vi "DAQ.Create DAQmx Asynch Read.vi"(8 "error in (no error)":errorcluster, 11 "Array":refnum<k21>[](array[refnum])) -> (0 "error out":errorcluster, 3 "VI out":refnum<vi>)   [LabVIEW 2019, in "Instrument.Lockin.lvlib" / "Instrument.DAQ.lvclass"]
uses:
  Instrument.DAQ.lvclass
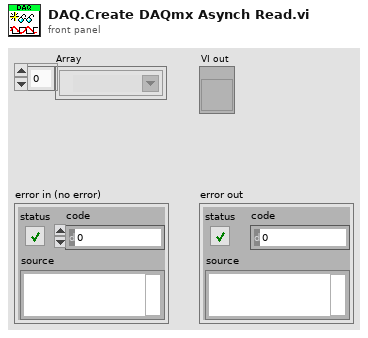
[diagram p1: front panel]
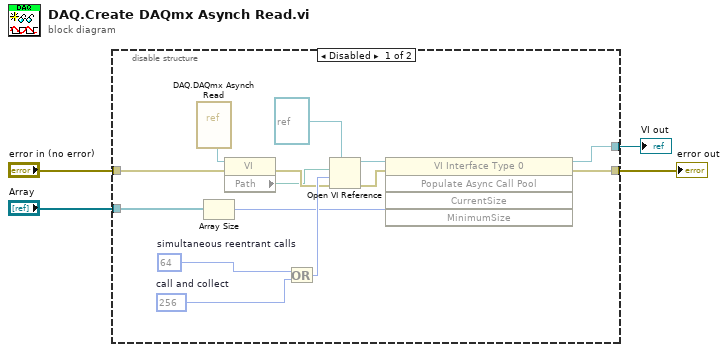
[diagram p0: block diagram]
diagram:
  n1 = disable-structure shown="Disabled" {
    disable-tunnel: "Array" -> [w8 _]
    disable-tunnel: [w7 _] -> w3
    disable-tunnel: [w6 w19] -> w2
    disable-tunnel: "error in (no error)" -> [w5 w19]
    frame Disabled {
      w16 = 64  # simultaneous reentrant calls
      w18 = 256  # call and collect
      n2 = vi-ref "DAQ.DAQmx Asynch Read.vi"() -> (w14:refnum<vi>)
      n3 = Array Size(array=w8) -> (size(s)=w15:i32)
      n4 = property class="VI"(reference=w14, error in=w5) -> (error out=w10:errorcluster, "Path"=w9:path)  [unwired: 1 out]
      n5 = Or(x=w16, y=w18) -> (x .or. y?=w17:i32)
      n6 = Open VI Reference(type specifier VI Refnum (for type only)=refnum<vi> refnum, vi path=w9, options=w17, error in (no error)=w10) -> (vi reference=w12:refnum<vi>, error out=w13:errorcluster)  [unwired: 2 in]
      n7 = invoke class="VI Interface Type 0" method="Populate Async Call Pool"(reference=w12, error in=w13, "MinimumSize"=w15) -> (reference out=w7:refnum<vi>, error out=w6:errorcluster)  [unwired: 2 in, 3 out]
    }
    frame Enabled {
    }
  }
  "VI out" <- w3
  "error out" <- w2
